vi "ManipulatorMotorControl.vi"   [LabVIEW 2015]
uses:
  Utilities/MotorPositionGlobals.vi
types:
  T1 = typedef "WPI_MotorControlDeviceRef.ctl" = cluster{"DeviceStatus":errorcluster, "Type":T2, "PWM":cluster{"PWM Channel":T3, "DeadBand":T4}, "CAN":cluster{"Device Number":u8, "Control Mode":T5, "Semaphore":T6, "Max Vout":dbl, "TalonSRX Control Mode":T7}, "Invert":bool}
  T2 = typedef "WPI_MotorControlType.ctl" = enum16{"PWM", "CAN", "CANTalonSRX"}
  T3 = typedef "FPGA_DIOPWMChannel.ctl" = enum8{"PWM 0", "PWM 1", "PWM 2", "PWM 3", "PWM 4", "PWM 5", "PWM 6", "PWM 7", "PWM 8", "PWM 9", "PWM MXP 0", "PWM MXP 1", "PWM MXP 2", "PWM MXP 3", "PWM MXP 4", "PWM MXP 5", "PWM MXP 6", "PWM MXP 7", "PWM MXP 8", "PWM MXP 9", "Invalid"}
  T4 = typedef "WPI_PWMDeadband.ctl" = cluster{"Name":string, "maxPositivePwm":i32, "minPositivePwm":i32, "centerPwm":i32, "maxNegativePwm":i32, "minNegativePwm":i32, "angularRange":u16}
  T5 = typedef "WPI_CANJaguar_ControlMode.ctl" = enum8{"Percent VBus", "Current", "Speed", "Position", "Voltage"}
  T6 = typedef "Semaphore RefNum" = refnum<k1>
  T7 = typedef "WPI_CANTalonSRX_APIControlMode.ctl" = enum8{"Percent VBus", "Speed", "Position", "Slave", "Unchanged / Invalid", "Voltage Compensation", "Current", "Motion Profile"}
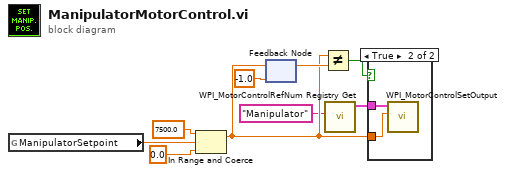
[diagram p0: block diagram]
diagram:
  n1 = global read "MotorPositionGlobals.vi" "ManipulatorSetpoint"() -> (w3:dbl)
  n2 = In Range and Coerce(upper limit=7500.0, x=w3, lower limit=0.0) -> (coerced(x)=w5:dbl)  [unwired: 1 out]
  n3 = feedback-in #1(w5) -> ()
  n4 = feedback #1(-1.0 ("upper limit")) -> (w6:dbl)
  n5 = Not Equal?(x=w5, y=w6) -> (x != y?=w4:bool)
  n6 = call <vilib>:"WPI_MotorControlRefNum Registry Get.vi"("refnum name"="Manipulator") -> ("MotorControlDevRef"=w1:T1)  [unwired: 9 in, 1 out]
  n7 = case shown="True" w4 {
    tunnel: w1 -> [_ w11]
    tunnel: w5 -> [_ w10]
    frame False {
    }
    frame True {
      n8 = call <vilib>:"WPI_MotorControlSetOutput.vi"("Output"=w10, "MotorControlDevRef"=w11) -> ()  [unwired: 7 in, 3 out]
    }
  }
